vi "ContourPlot v3.1-IV.vi"() -> ()   [LabVIEW 2019]
uses:
  <vilib>/Utility/file.llb/Read Delimited Spreadsheet (DBL).vi
  <vilib>/gmath/NI_Gmath.lvlib
panel:
  in  "V divide I":bool
  in  "Begin":i32=1000
  in  "length":i32=1000
  in  "Contact Resistance":dbl
  out "Ready?":bool=TRUE
  in  "Auto x axis T":bool=TRUE
  in  "Tab Control 2":enum32{"Contour", "Curve"}(tab)
  out "Intensity Graph":dbl[][](graph)
  out "XY Graph":cluster{"Y":dbl[], "Y":dbl[]}[](graph)=[{"Y"=[0.0, 0.1, 0.2, 0.30000000000000004, 0.4, 0.5, 0.6000000000000001, 0.7000000000000001, 0.8, 0.9, 1.0, 1.1, 1.2000000000000002, 1.3, 1.4000000000000001, 1.5, 1.6, 1.7000000000000002, 1.8, 1.9000000000000001, 2.0, 2.1, 2.2, 2.3000000000000003, 2.4000000000000004, 2.5, 2.6, 2.7, 2.8000000000000003, 2.9000000000000004, 3.0, 3.1, 3.2, 3.3000000000000003, 3.4000000000000004, 3.5, 3.6, 3.7, 3.8000000000000003, 3.9000000000000004, 4.0, 4.1000000000000005, 4.2, 4.3, 4.4, 4.5, 4.6000000000000005, 4.7, 4.800000000000001, 4.9, 5.0, 5.1000000000000005, 5.2, 5.300000000000001, 5.4, 5.5, 5.6000000000000005, 5.7, 5.800000000000001, 5.9, 6.0, 6.1000000000000005, 6.2, 6.300000000000001, 6.4, 6.5, 6.6000000000000005, 6.7, 6.800000000000001, 6.9, 7.0, 7.1000000000000005, 7.2, 7.300000000000001, 7.4, 7.5, 7.6000000000000005, 7.7, 7.800000000000001, 7.9, 8.0, 8.1, 8.200000000000001, 8.3, 8.4, 8.5, 8.6, 8.700000000000001, 8.8, 8.9, 9.0, 9.1, 9.200000000000001, 9.3, 9.4, 9.5, 9.600000000000001, 9.700000000000001, 9.8, 9.9, 10.0, 10.100000000000001, 10.200000000000001, 10.3, 10.4, 10.5, 10.600000000000001, 10.700000000000001, 10.8, 10.9, 11.0, 11.100000000000001, 11.200000000000001, 11.3, 11.4, 11.5, 11.600000000000001, 11.700000000000001, 11.8, 11.9], "Y"=[0.0, 0.0, 0.0, 0.0, 0.0, 0.0, 0.0, 0.0, 0.0, 0.0, nan, 0.0, 0.0, 0.0, 0.0, 0.0, 0.0, 0.0, 0.0, 0.0, 0.0, 0.0, 0.0, 0.0, 0.0, 0.0, 0.0, 0.0, 0.0, 0.0, 0.0, 0.0, 0.0, 0.0, 0.0, 0.0, 0.0, 0.0, 0.0, 0.0, 0.0, 0.0, 0.0, 0.0, 0.0, 0.0, 0.0, 0.0, nan, 0.0, 0.0, 0.0, 0.0, 0.0, 0.0, 0.0, 0.0, 0.0, 0.0, 0.0, 0.0, 0.0, 0.0, 0.0, 0.0, 0.0, 0.0, 0.0, 0.0, 0.0, 0.0, 0.0, 0.0, 0.0, 0.0, 0.0, 0.0, 0.0, 0.0, 0.0, 0.0, 0.0, 0.0, 0.0, 0.0, 0.0, 0.0, 0.0, 0.0, 0.0, 0.0, 0.0, 0.0, 0.0, 0.0, 0.0, 0.0, 0.0, 0.0, 0.0, 0.0, 0.0, nan, 0.0, 0.0, 0.0, 0.0, 0.0, 0.0, 0.0, nan, 0.0, 0.0, 0.0, 0.0, 0.0, 0.0, 0.0, 0.0, 0.0]}]
  in  "Voltage treshold":dbl=1.2e-05 format="%_3g"
  in  "Ignore points":i32=250
  in  "Tab Control":enum32{"IV"}(tab)
  out "IV":cluster{dbl[], "Intensity Graph":dbl[]}(graph)
  in  "book number":i32=414
  in  "file path (dialog if empty)":path=path "C:/Users/gyue/Box/Guang Yue uiuc research box folder/data/Contour plot"
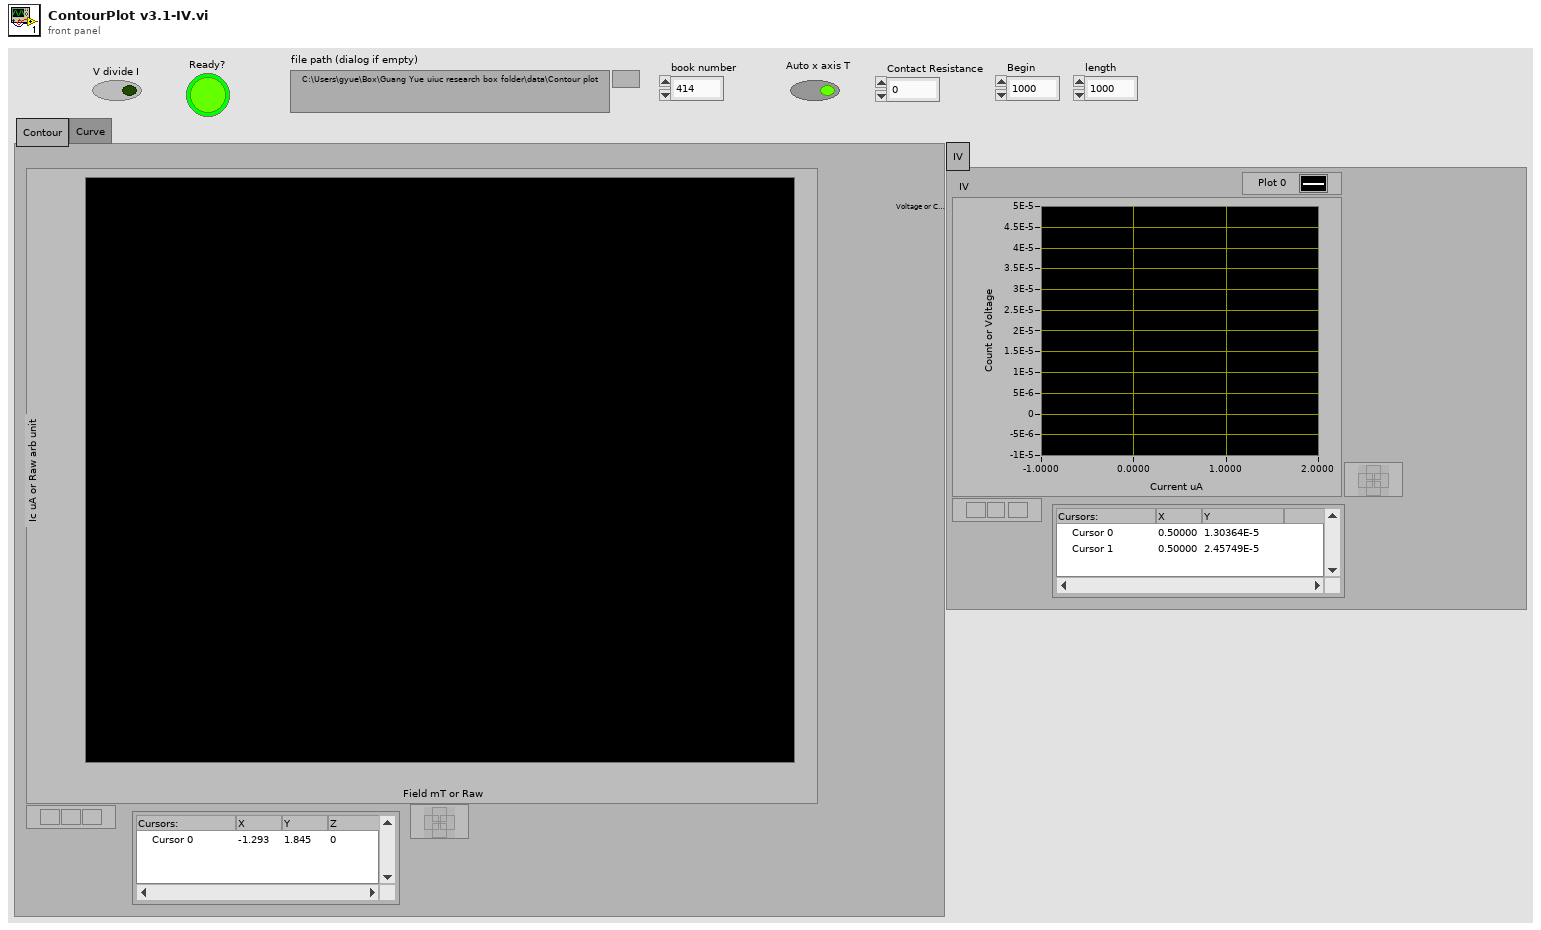
[diagram p1: front panel]
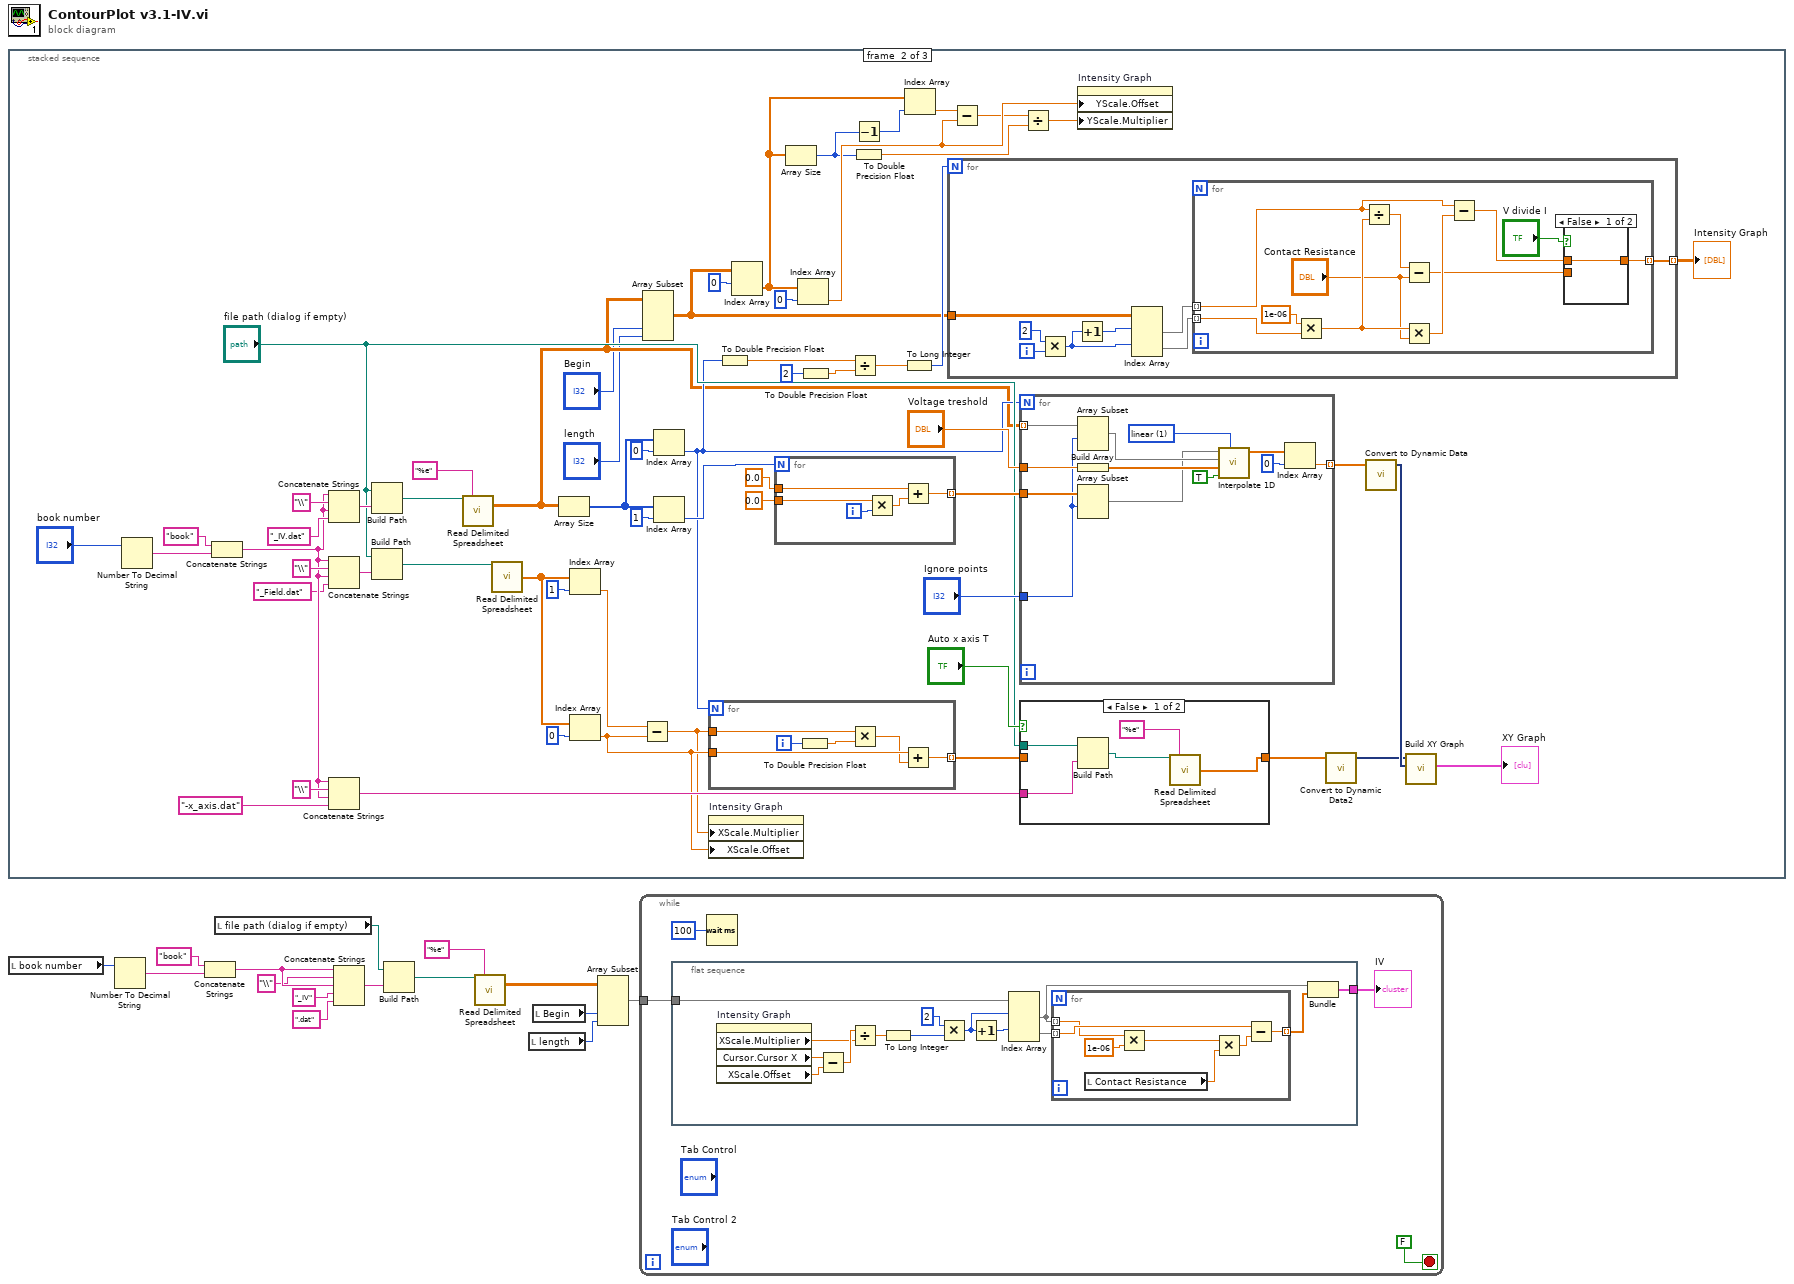
[diagram p0: block diagram]
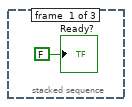
[diagram p2: hidden frame]
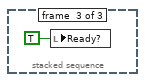
[diagram p5: hidden frame]
diagram:
  n1 = stacked-sequence {
    frame #0 {
      "Ready?" <- FALSE ("Ready?")
    }
    frame #1 {
      n2 = Number To Decimal String(number="book number") -> (decimal integer string=w72:string)  [unwired: 1 in]
      n3 = Concatenate Strings("book" ("string"), w72) -> (w45:string)
      n4 = Concatenate Strings(w45, "\\" ("string"), w45, "_IV.dat" ("string")) -> (w73:string)
      n5 = Concatenate Strings(w45, "\\" ("string"), w45, "_Field.dat" ("string")) -> (w74:string)
      n6 = Concatenate Strings(w45, "\\" ("string"), w45, "-x_axis.dat" ("string")) -> (w52:string)
      n7 = Build Path(base path="file path (dialog if empty)", name or relative path=w73) -> (appended path=w76:path)
      n8 = Build Path(base path="file path (dialog if empty)", name or relative path=w74) -> (appended path=w75:path)
      n9 = call-poly <vilib>:"Read Delimited Spreadsheet.vi"("file path (dialog if empty)"=w76, "format (%.3f)"="%e") -> ("all rows"=w34:dbl[][])  [unwired: 8 in, 5 out]
      n10 = call-poly <vilib>:"Read Delimited Spreadsheet.vi"("file path (dialog if empty)"=w75) -> ("first row"=w31:dbl[])  [unwired: 9 in, 5 out]
      n11 = Array Size(array=w34) -> (size(s)=w51:i32[])
      n12 = Index Array(array=w31, index=1 ("index (row)")) -> (element=w30:dbl)
      n13 = Index Array(array=w31, index=0 ("index (row)")) -> (element=w29:dbl)
      n14 = Subtract(x=w30, y=w29) -> (x-y=w28:dbl)
      n15 = Array Subset(array=w34, index (col)="Begin", length (col)="length") -> (w27:dbl[][])  [unwired: 2 in]
      n16 = Index Array(array=w51, index=0) -> (element=w41:i32)
      n17 = Index Array(array=w51, index=1) -> (element=w49:i32)
      n18 = for {
        N: w41 -> [_]
        tunnel: w29 -> [w109]
        tunnel: w28 -> [w107]
        tunnel: [w105] -> w57 mode=indexing
        i -> [w108]
        n19 = To Double Precision Float(number=w108) -> (double precision float=w104:dbl)
        n20 = Multiply(x=w107, y=w104) -> (x*y=w106:dbl)
        n21 = Add(x=w109, y=w106) -> (x+y=w105:dbl)
      }
      n22 = property on="Intensity Graph" class="IntGraph (strict)"("XScale.Multiplier"=w28, "XScale.Offset"=w29) -> ()  [unwired: 2 in, 2 out]
      n23 = To Double Precision Float(number=w41) -> (double precision float=w39:dbl)
      n24 = Index Array(array=w27, index (row)=0) -> (element=w24:dbl[])  [unwired: 1 in]
      n25 = for {
        N: w49 -> [_]
        tunnel: 0.0 ("Numeric") -> [w114]
        tunnel: 0.0 ("Numeric") -> [w112]
        tunnel: [w110] -> w59 mode=indexing
        i -> [w113]
        n26 = Multiply(x=w112, y=w113) -> (x*y=w111:dbl)
        n27 = Add(x=w114, y=w111) -> (x+y=w110:dbl)
      }
      n28 = Array Size(array=w24) -> (size(s)=w19:i32)
      n29 = Index Array(array=w24, index=0) -> (element=w21:dbl)
      n30 = To Double Precision Float(number=2 ("y")) -> (double precision float=w38:dbl)
      n31 = Divide(x=w39, y=w38) -> (x/y=w37:dbl)
      n32 = Decrement(x=w19) -> (x-1=w23:i32)
      n33 = To Double Precision Float(number=w19) -> (double precision float=w18:dbl)
      n34 = To Long Integer(number=w37) -> (32bit integer=w36:i32)
      n35 = Index Array(array=w24, index=w23) -> (element=w22:dbl)
      n36 = for {
        N: w36 -> [_]
        tunnel: w27 -> [w82]
        tunnel: [w77] -> w35 mode=indexing
        i -> [w84]
        n37 = Multiply(x=2, y=w84) -> (x*y=w80:i32)
        n38 = Increment(x=w80) -> (x+1=w81:i32)
        n39 = Index Array(array=w82, index (row) #1=w81, index (row) #2=w80) -> (element #1=w79:dbl[], element #2=w78:dbl[])  [unwired: 2 in]
        n40 = for {
          tunnel: w79 -> [w92] mode=indexing
          tunnel: w78 -> [w95] mode=indexing
          tunnel: [w89] -> w77 mode=indexing
          n41 = Multiply(x=1e-06, y=w95) -> (x*y=w91:dbl)
          n42 = Divide(x=w92, y=w91) -> (x/y=w88:dbl)
          n43 = Subtract(x=w88, y="Contact Resistance") -> (x-y=w86:dbl)
          n44 = Multiply(x=w91, y="Contact Resistance") -> (x*y=w94:dbl)
          n45 = Subtract(x=w92, y=w94) -> (x-y=w87:dbl)
          n46 = case shown="False" "V divide I" {
            tunnel: w86 -> [_ w97]
            tunnel: [w96 w97] -> w89
            tunnel: w87 -> [w96 _]
            frame False {
            }
            frame True {
            }
          }
        }
      }
      "Intensity Graph" <- w35
      n47 = Subtract(x=w22, y=w21) -> (x-y=w20:dbl)
      n48 = for {
        N: w41 -> [_]
        tunnel: w34 -> [w119] mode=indexing
        tunnel: w59 -> [w120]
        tunnel: [w121] -> w65 mode=indexing
        tunnel: "Ignore points" -> [w115]
        tunnel: "Voltage treshold" -> [w116]
        w125 = 1 items=["nearest", "linear", "spline", "cubic Hermite", "Lagrange"] ("method")
        n49 = Array Subset(array=w119, index=w115) -> (w118:dbl[])  [unwired: 1 in]
        n50 = Build Array(w116) -> (w124:dbl[])
        n51 = Array Subset(array=w120, index=w115) -> (w117:dbl[])  [unwired: 1 in]
        n52 = call <vilib>:"Interpolate 1D.vi"("method"=w125, "X is monotonic"=TRUE, "xi"=w124, "X"=w118, "Y"=w117) -> ("yi"=w123:dbl[])  [unwired: 4 in, 2 out]
        n53 = Index Array(array=w123, index=0) -> (element=w121:dbl)
      }
      n54 = case shown="False" "Auto x axis T" {
        tunnel: w57 -> [_ w103]
        tunnel: [w98 w103] -> w56
        tunnel: "file path (dialog if empty)" -> [w102 _]
        tunnel: w52 -> [w101 _]
        frame False {
          n55 = Build Path(base path=w102, name or relative path=w101) -> (appended path=w100:path)
          n56 = call-poly <vilib>:"Read Delimited Spreadsheet.vi"("file path (dialog if empty)"=w100, "format (%.3f)"="%e") -> ("first row"=w98:dbl[])  [unwired: 8 in, 5 out]
        }
        frame True {
        }
      }
      n57 = Divide(x=w20, y=w18) -> (x/y=w17:dbl)
      n58 = property on="Intensity Graph" class="IntGraph (strict)"("YScale.Offset"=w21, "YScale.Multiplier"=w17) -> ()  [unwired: 2 in, 2 out]
      n59 = call "Convert to Dynamic Data2"("Array"=w56) -> ("Dynamic Data Type"=w63:dynamicdata)  [unwired: 3 in]
      n60 = call "Convert to Dynamic Data"("Array"=w65) -> ("Dynamic Data Type"=w64:dynamicdata)  [unwired: 3 in]
      n61 = call "Build XY Graph"("Y Input"=w64, "X Input"=w63) -> ("XY Graph"=→"XY Graph":cluster{"X":dbl[], "Y":dbl[]}[])  [unwired: 8 in, 1 out]
    }
    frame #2 {
      n62 = local write "Ready?"(TRUE ("Ready?")) -> ()
    }
  }
  n63 = local read "book number"() -> (w15:i32)
  n64 = Number To Decimal String(number=w15) -> (decimal integer string=w6:string)  [unwired: 1 in]
  n65 = Concatenate Strings("book" ("string"), w6) -> (w12:string)
  n66 = local read "file path (dialog if empty)"() -> (w5:path)
  n67 = Concatenate Strings(w12, "\\" ("string"), w12, "_IV" ("string"), ".dat" ("string")) -> (w13:string)
  n68 = Build Path(base path=w5, name or relative path=w13) -> (appended path=w14:path)
  n69 = call-poly <vilib>:"Read Delimited Spreadsheet.vi"("file path (dialog if empty)"=w14, "format (%.3f)"="%e") -> ("all rows"=w4:dbl[][])  [unwired: 8 in, 5 out]
  n70 = local read "length"() -> (w3:i32)
  n71 = local read "Begin"() -> (w1:i32)
  n72 = Array Subset(array=w4, index (col)=w1, length (col)=w3) -> (w2:dbl[][])  [unwired: 2 in]
  n73 = while {
    tunnel: w2 -> [w128]
    stop <- FALSE stop-if-true
    n74 = flat-sequence {
      tunnel: [w141] -> w131
      tunnel: w128 -> [w138]
      frame #0 {
        n75 = property on="Intensity Graph" class="IntGraph (strict)"() -> ("XScale.Multiplier"=w144:dbl, "Cursor.Cursor X"=w143:dbl, "XScale.Offset"=w142:dbl)  [unwired: 2 in, 2 out]
        n76 = Subtract(x=w143, y=w142) -> (x-y=w145:dbl)
        n77 = Divide(x=w145, y=w144) -> (x/y=w140:dbl)
        n78 = To Long Integer(number=w140) -> (32bit integer=w135:i32)
        n79 = Multiply(x=2, y=w135) -> (x*y=w137:i32)
        n80 = Increment(x=w137) -> (x+1=w136:i32)
        n81 = Index Array(array=w138, index (row) #1=w137, index (row) #2=w136) -> (element #1=w132:dbl[], element #2=w134:dbl[])  [unwired: 2 in]
        n82 = for {
          tunnel: w134 -> [w152] mode=indexing
          tunnel: w132 -> [w151] mode=indexing
          tunnel: [w149] -> w133 mode=indexing
          n83 = local read "Contact Resistance"() -> (w148:dbl)
          n84 = Multiply(x=w151, y=1e-06 ("x")) -> (x*y=w147:dbl)
          n85 = Multiply(x=w147, y=w148) -> (x*y=w150:dbl)
          n86 = Subtract(x=w152, y=w150) -> (x-y=w149:dbl)
        }
        n87 = Bundle(w132, w133) -> (w141:cluster{dbl[], dbl[]})  [unwired: 1 in]
      }
    }
    n88 = Wait (ms)(milliseconds to wait=u32 100) -> ()  [unwired: 1 out]
    "IV" <- w131
  }
